vi "Set Encodings.vi"(6 "Encodings [UTF-8, UCS-16]":refnum<class "CConfig Encoding.lvclass">[](array[class])=[refnum, refnum], 8 "error in (no error)":errorcluster, 11 "Encoding in":refnum<class "CConfig Automatic Encoding.lvclass">) -> (0 "error out":errorcluster, 3 "Encoding out":refnum<class "CConfig Automatic Encoding.lvclass">)   [LabVIEW 2013, in "CConfig Automatic Encoding.lvclass"]
doc: "Copyright 2018, Carya Automatisering, Wiebe Walstra."
uses:
  CConfig Automatic Encoding.lvclass
  CConfig Encoding.lvclass
  CConfig UTF-8-BOM Encoding/CConfig UTF-8-BOM Encoding.lvclass
  CConfig UCS-16 Encoding/CConfig UCS-16 Encoding.lvclass
  CConfig Automatic Encoding.lvclass/CConfig Automatic Encoding.ctl
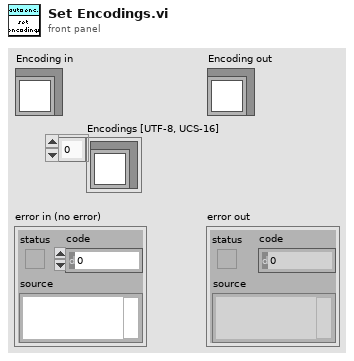
[diagram p1: front panel]
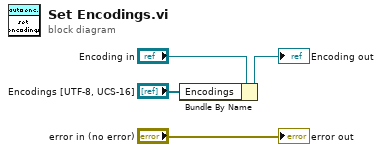
[diagram p0: block diagram]
diagram:
  n1 = Bundle By Name(cluster="Encoding in", "Encodings"="Encodings [UTF-8, UCS-16]") -> (→"Encoding out":refnum<class "CConfig Automatic Encoding.lvclass">)
  "error out" <- "error in (no error)"
